vi "Calculate Motor Encoders.vi"(8 "error in (no error)":errorcluster, 10 "color change":dbl, 11 "Control Panel in":refnum<class "Control Panel.lvclass">) -> (0 "error out":errorcluster, 2 "Encoder Ticks":dbl, 3 "Control Panel out":refnum<class "Control Panel.lvclass">)   [LabVIEW 2019, in "Control Panel.lvlib" / "Control Panel.lvclass"]
uses:
  Control Panel.lvclass
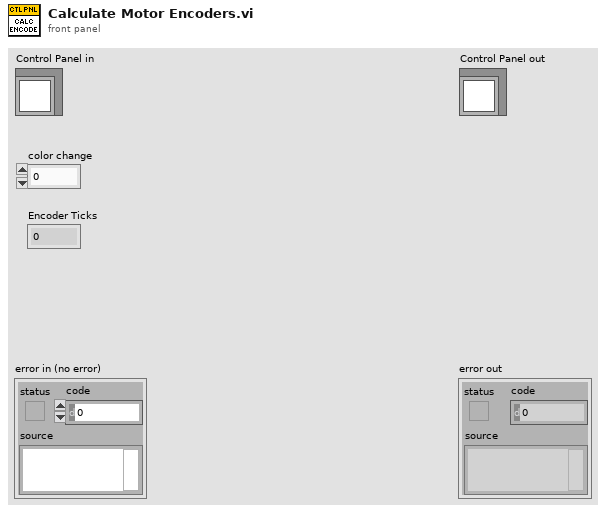
[diagram p1: front panel]
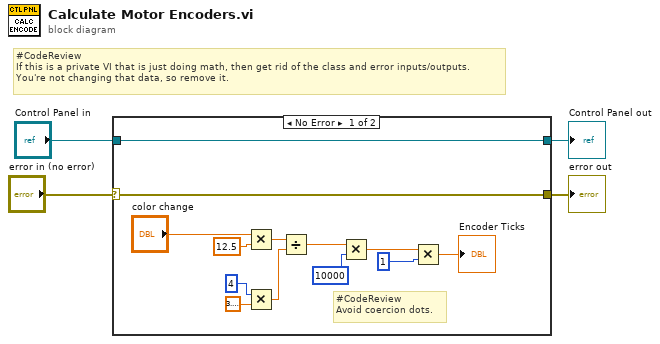
[diagram p0: block diagram]
diagram:
  # "#CodeReview\nIf this is a private VI that is just doing math, then get rid of the class and error inputs/outputs.\nYou're not changing that data, so remove it."
  n1 = case shown="No Error" "error in (no error)" {
    selector: "error in (no error)" -> [w16 w19]
    tunnel: [w16 w19] -> w3
    tunnel: [w17 w18] -> w1
    tunnel: "Control Panel in" -> [w17 w18]
    frame No Error {
      # "#CodeReview\nAvoid coercion dots."
      n2 = Multiply(x="color change", y=12.5) -> (x*y=w13:dbl)
      n3 = Multiply(x=4, y=3.141592653589793) -> (x*y=w10:dbl)
      n4 = Divide(x=w13, y=w10) -> (x/y=w9:dbl)
      n5 = Multiply(x=w9, y=10000) -> (x*y=w7:dbl)
      n6 = Multiply(x=w7, y=1) -> (x*y=→"Encoder Ticks":dbl)
    }
    frame Error {
    }
  }
  "error out" <- w3
  "Control Panel out" <- w1
